vi "Save Repos to File.vi"(8 "error in":errorcluster, 11 "Repos":refnum<class "Repo.lvclass">[](array[class])) -> (0 "error out":errorcluster, 3 "Repos dup":refnum<class "Repo.lvclass">[](array[class]))   [LabVIEW 2020, in "WSsupport.lvlib"]
uses:
  WSsupport.lvlib
  Packages/Repo_class/Repo.lvclass
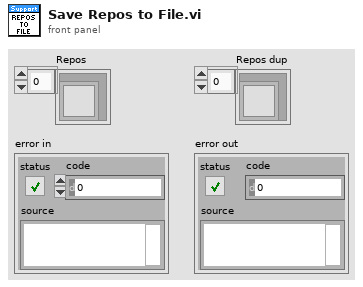
[diagram p1: front panel]
types:
  T1 = enum16{"open", "replace", "create", "open or create", "replace or create", "replace or create with confirmation"}
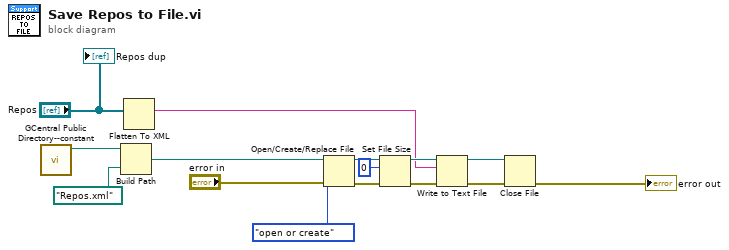
[diagram p0: block diagram]
diagram:
  n1 = call "GCentral Public Directory--constant.vi"() -> ("GCentral Public Dir"=w15:path)  [unwired: 11 in]
  n2 = Build Path(base path=w15, name or relative path=path "Repos.xml") -> (appended path=w13:path)
  n3 = Flatten To XML(6:"Repos") -> (2:w1:string)
  n4 = Open/Create/Replace File(file path (use dialog)=w13, error in="error in", operation (0:open)=T1."open or create") -> (refnum out=w4:refnum<file>, error out=w11:errorcluster)  [unwired: 3 in, 1 out]
  n5 = Set File Size(4:w11, 6:i64 0 ("size (in bytes)"), 7:w4) -> (0:w5:errorcluster, 3:w3:refnum<file>)
  n6 = Write to Text File(file (use dialog)=w3, text=w1, error in=w5) -> (refnum out=w10:refnum<file>, error out=w9:errorcluster)  [unwired: 1 in, 1 out]
  n7 = Close File(refnum=w10, error in=w9) -> (error out=→"error out":errorcluster)  [unwired: 1 out]
  "Repos dup" <- "Repos"
